vi "Test.vi"() -> ()   [LabVIEW 2018, in "Application.lvlib" / "Dictionary.lvclass"]
uses:
  Dictionary.lvclass
  Dictionary.lvclass/Dictionary.ctl
  99283ed1-40a4-4449-ae42-fb7129a125c0.vi
  Get Data DVR.vi
panel:
  out "Value":variant
  out "Keys":string[](array[string])
  out "x-y 2":dbl format="%^#_6e"
  out "Values":variant[](array[variant])
  out "x-y":dbl format="%^#_6e"
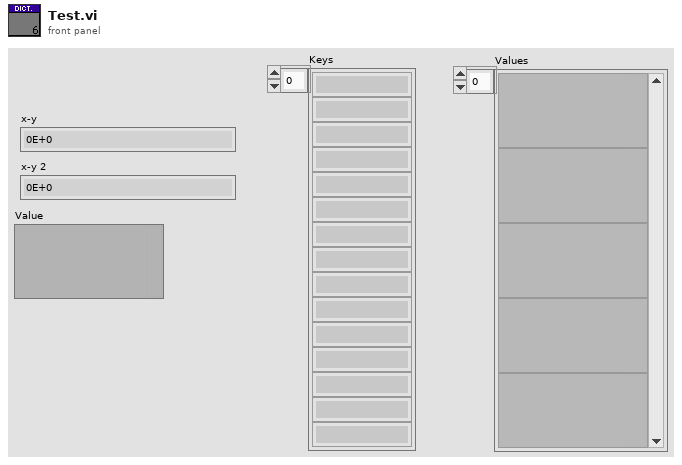
[diagram p1: front panel]
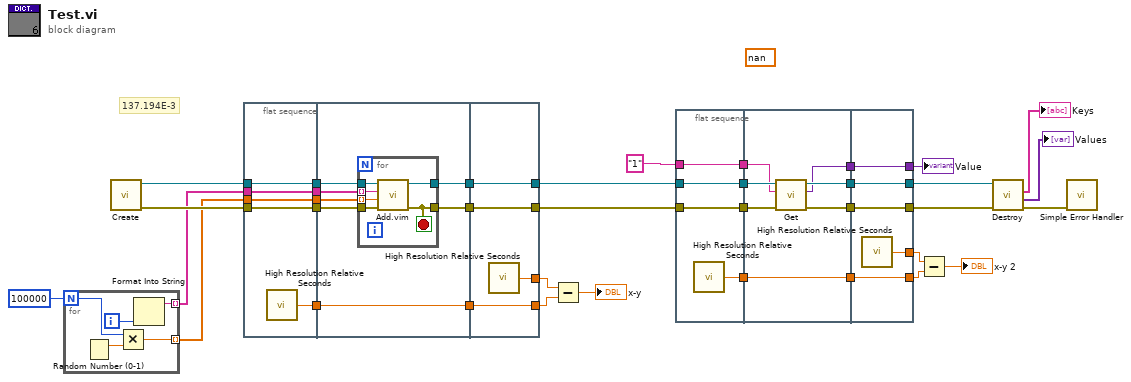
[diagram p0: block diagram]
diagram:
  (unwired) nan ("x*y")
  # "137.194E-3"
  n1 = for {
    N: 100000 -> [w41]
    tunnel: [w39] -> w33 mode=indexing
    tunnel: [w37] -> w32 mode=indexing
    i -> [w38]
    n2 = Random Number (0-1)() -> (number: 0 to 1=w40:dbl)
    n3 = Multiply(x=w41, y=w40) -> (x*y=w39:dbl)
    n4 = Format Into String(w38) -> (resulting string=w37:string)  [unwired: 3 in, 1 out]
  }
  n5 = call "Create.vi"() -> ("error out"=w35:errorcluster, "Dictionary out"=w34:refnum<class "Dictionary.lvclass">)  [unwired: 10 in]
  n6 = flat-sequence {
    tunnel: w32 -> [w43]
    tunnel: w33 -> [w44]
    tunnel: w34 -> [w45]
    tunnel: w35 -> [w46]
    tunnel: [w46] -> w31
    tunnel: [w45] -> w30
    tunnel: [w44] -> w29
    tunnel: [w43] -> w28
    tunnel: [w42] -> w24
    tunnel: w31 -> [w53]
    tunnel: w30 -> [w52]
    tunnel: w29 -> [w51]
    tunnel: w28 -> [w50]
    tunnel: [w49] -> w27
    tunnel: [w48] -> w26
    tunnel: [w47] -> w25
    tunnel: w24 -> [w47]
    tunnel: [w62] -> w10
    tunnel: [w63] -> w11
    tunnel: w27 -> [w63]
    tunnel: w26 -> [w62]
    tunnel: [w61] -> w22
    tunnel: w25 -> [w61]
    tunnel: [w60] -> w23
    frame #0 {
      n7 = call <vilib>:"High Resolution Relative Seconds.vi"() -> ("relative seconds"=w42:dbl)
    }
    frame #1 {
      n8 = for {
        tunnel: w53 -> [w58]
        tunnel: w52 -> [w59]
        tunnel: w51 -> [w55] mode=indexing
        tunnel: w50 -> [w56] mode=indexing
        tunnel: [w54] -> w49
        tunnel: [w57] -> w48
        stop <- w57 stop-if-true
        n9 = call "Add.vim"("error in (no error)"=w58, "Value"=w55, "Key"=w56, "Dictionary in"=w59) -> ("error out"=w57:errorcluster, "Dictionary out"=w54:refnum<class "Dictionary.lvclass">)  [unwired: 5 in, 1 out]
      }
    }
    frame #2 {
      n10 = call <vilib>:"High Resolution Relative Seconds.vi"() -> ("relative seconds"=w60:dbl)
    }
  }
  n11 = Subtract(x=w23, y=w22) -> (x-y=→"x-y":dbl)
  n12 = flat-sequence {
    tunnel: w10 -> [w66]
    tunnel: w11 -> [w67]
    tunnel: [w67] -> w19
    tunnel: [w66] -> w18
    tunnel: [w65] -> w17
    tunnel: "1" -> [w64]
    tunnel: [w64] -> w16
    tunnel: w19 -> [w73]
    tunnel: w18 -> [w72]
    tunnel: w17 -> [w74]
    tunnel: [w71] -> w15
    tunnel: [w70] -> w14
    tunnel: [w74] -> w13
    tunnel: w16 -> [w68]
    tunnel: [w69] -> w12
    tunnel: [w77] -> w3
    tunnel: [w78] -> w8
    tunnel: [w79] -> w7
    tunnel: w15 -> [w79]
    tunnel: w14 -> [w78]
    tunnel: w13 -> [w77]
    tunnel: [w76] -> w4
    tunnel: w12 -> [w75]
    tunnel: [w75] -> w1
    frame #0 {
      n13 = call <vilib>:"High Resolution Relative Seconds.vi"() -> ("relative seconds"=w65:dbl)
    }
    frame #1 {
      n14 = call "Get.vi"("error in (no error)"=w72, "Key"=w68, "Dictionary in"=w73) -> ("error out"=w71:errorcluster, "Value"=w69:variant, "Dictionary out"=w70:refnum<class "Dictionary.lvclass">)  [unwired: 5 in, 1 out]
    }
    frame #2 {
      n15 = call <vilib>:"High Resolution Relative Seconds.vi"() -> ("relative seconds"=w76:dbl)
    }
  }
  n16 = Subtract(x=w4, y=w3) -> (x-y=→"x-y 2":dbl)
  n17 = call "Destroy.vi"("error in (no error)"=w7, "Dictionary in"=w8) -> ("error out"=w5:errorcluster, "Values"=→"Values":variant[], "Keys"=→"Keys":string[])  [unwired: 7 in]
  n18 = call <vilib>:"Simple Error Handler.vi"("error in (no error)"=w5) -> ()  [unwired: 4 in, 5 out]
  "Value" <- w1
